vi "Climb Initialize.vi"(6 "Skywalker name":string="Skywalker", 8 "Skywalker ID":u8, 9 "Climber name":string="Climb Motor", 10 "Climber Slave":u8, 11 "CLimber Master":u8) -> ()   [LabVIEW 2019]
uses:
  <vilib>/Rock Robotics/WPI/ThirdParty/Phoenix-LabVIEW/Motor Controller/Controls/CTRE_Phoenix_MotorControl_LimitSwitchSource_Local.ctl
  <vilib>/Rock Robotics/WPI/ThirdParty/Phoenix-LabVIEW/Motor Controller/Controls/CTRE_Phoenix_MotorControl_LimitSwitchNormal.ctl
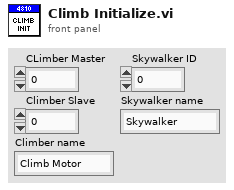
[diagram p1: front panel]
types:
  T1 = typedef "CTRE_Phoenix_MotorControl_LimitSwitchNormal.ctl" = enum16{"Normally Open", "Normally Closed", "Disabled"}
  T2 = typedef "CTRE_Phoenix_MotorControl_LimitSwitchSource_Local.ctl" = enum16{"Feedback Connector", "Remote Talon SRX", "Remote CANifier", "Deactivated"}
  T3 = enum16{"FollowerType_PercentOutput", "FollowerType_AuxOutput1"}
  T4 = typedef "WPI_MotorControlDeviceRef.ctl" = cluster{"DeviceStatus":errorcluster, "Type":T5, "PWM":cluster{"PWM Channel":T6, "DeadBand":T7}, "CAN":cluster{"Device Number":u8, "SetOutput VI Ref":variant, "GetOutput VI Ref":variant, "Enable VI Ref":variant, "Disable VI Ref":variant, "Data":variant}, "Invert":bool, "DIO PWM":cluster{"PWM \"Enable\" Channel":T6, "DIOChannel":T8, "PWM Rate":dbl}}
  T5 = typedef "WPI_MotorControlType.ctl" = enum16{"PWM", "CAN", "DIO PWM"}
  T6 = typedef "FPGA_DIOPWMChannel.ctl" = enum8{"PWM 0", "PWM 1", "PWM 2", "PWM 3", "PWM 4", "PWM 5", "PWM 6", "PWM 7", "PWM 8", "PWM 9", "PWM MXP 0", "PWM MXP 1", "PWM MXP 2", "PWM MXP 3", "PWM MXP 4", "PWM MXP 5", "PWM MXP 6", "PWM MXP 7", "PWM MXP 8", "PWM MXP 9", "Invalid"}
  T7 = typedef "WPI_PWMDeadband.ctl" = cluster{"Name":string, "maxPositivePwm":i32, "minPositivePwm":i32, "centerPwm":i32, "maxNegativePwm":i32, "minNegativePwm":i32, "angularRange":u16}
  T8 = typedef "FPGA_DIOChannel.ctl" = enum8{"DIO 0", "DIO 1", "DIO 2", "DIO 3", "DIO 4", "DIO 5", "DIO 6", "DIO 7", "DIO 8", "DIO 9", "DIO MXP 0", "DIO MXP 1", "DIO MXP 2", "DIO MXP 3", "DIO MXP 4", "DIO MXP 5", "DIO MXP 6", "DIO MXP 7", "DIO MXP 8", "DIO MXP 9", "DIO MXP 10", "DIO MXP 11", "DIO MXP 12", "DIO MXP 13", "DIO MXP 14", "DIO MXP 15", "SPI Port CS1", "SPI Port CS2", "SPI Port CS3", "SPI Port MISO", "SPI Port MOSI", "Invalid"}
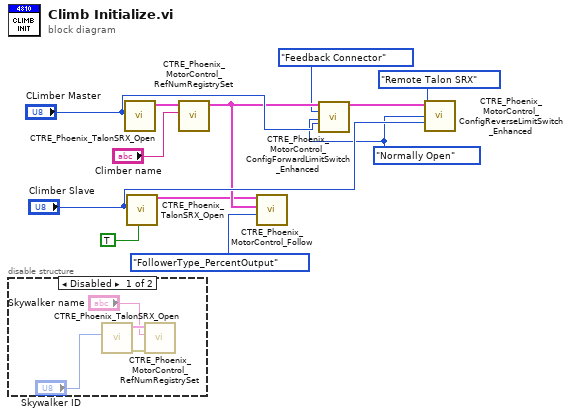
[diagram p0: block diagram]
diagram:
  w10 = CTRE_Phoenix_MotorControl_LimitSwitchNormal."Normally Open" ("NormallyOpenOrClosed")
  n1 = disable-structure shown="Disabled" {
    frame Disabled {
      n2 = call <vilib>:"CTRE_Phoenix_TalonSRX_Open.vi"("Device Number"="Skywalker ID") -> ("error out"=w16:errorcluster, "CAN Talon SRX Ref"=w15:T4)  [unwired: 9 in]
      n3 = call <vilib>:"CTRE_Phoenix_MotorControl_RefNumRegistrySet.vi"("error in (no error)"=w16, "refnum name"="Skywalker name", "PhoenixMotorControlDevRef"=w15) -> ()  [unwired: 7 in, 2 out]
    }
    frame Enabled {
    }
  }
  n4 = call <vilib>:"CTRE_Phoenix_TalonSRX_Open.vi"("Device Number"="CLimber Master") -> ("CAN Talon SRX Ref"=w1:T4)  [unwired: 9 in, 1 out]
  n5 = call <vilib>:"CTRE_Phoenix_TalonSRX_Open.vi"("Invert"=TRUE, "Device Number"="Climber Slave") -> ("CAN Talon SRX Ref"=w2:T4)  [unwired: 8 in, 1 out]
  n6 = call <vilib>:"CTRE_Phoenix_MotorControl_RefNumRegistrySet.vi"("refnum name"="Climber name", "PhoenixMotorControlDevRef"=w1) -> ("PhoenixMotorControlDevRef"=w9:T4)  [unwired: 8 in, 1 out]
  n7 = call <vilib>:"CTRE_Phoenix_MotorControl_Follow.vi"("FollowerType"=T3."FollowerType_PercentOutput", "Master Controller to Follow"=w9, "PhoenixMotorControlDevRef"=w2) -> ()  [unwired: 7 in, 2 out]
  n8 = call <vilib>:"CTRE_Phoenix_MotorControl_ConfigForwardLimitSwitch_Enhanced.vi"("PhoenixMotorControlDevRef"=w9, "Limit Switch Source"=CTRE_Phoenix_MotorControl_LimitSwitchSource_Local."Feedback Connector", "NormallyOpenOrClosed"=w10, "deviceID"="CLimber Master") -> ("PhoenixMotorControlDevRef"=w7:T4)  [unwired: 10 in, 1 out]
  n9 = call <vilib>:"CTRE_Phoenix_MotorControl_ConfigReverseLimitSwitch_Enhanced.vi"("PhoenixMotorControlDevRef"=w7, "Limit Switch Source"=CTRE_Phoenix_MotorControl_LimitSwitchSource_Local."Remote Talon SRX", "NormallyOpenOrClosed"=w10, "deviceID"="Climber Slave") -> ()  [unwired: 10 in, 2 out]
